vi "Write Serial Output Channel IO.vi"(0 "packet word":u8[](array[numeric]), 1 "reset":bool, 2 "resources":T1, 3 "filler valid":bool[](array[boolean]), 5 "end of packet":bool, 7 "generate packet":bool, 9 "input valid":bool, 11 "header valid":bool) -> (4 "ready to generate packet":bool, 6 "num packets in tx buffer":fxp<+,14,14>, 8 "num generated packets":u64, 14 "tready":bool)   [LabVIEW 2020, in "GettingStarted_Gen_148X_FPGA.lvlib"]
uses:
  GettingStarted_Gen_148X_FPGA.lvlib
  Types/Serial Output Channel Resources.ctl
  Common/Types/Serial Output Channel IO.ctl
  Common/Types/Serial Output Channel IO 32b.ctl
  Common/Types/Serial Output Channel IO 64b.ctl
  Common/Types/I2C IO.ctl
  Common/Types/Single Serial Channel Resources.ctl
  <vilib>/rvi/eio/common/nirviEmuTemplateMethod_errors.vi
  <instrlib>/_niInstr/Basic Elements/v1/FPGA/Private/Count Up U64.vi
  <instrlib>/_niInstr/Data Formatting/v1/FPGA/Private/Convert/U8 array to Boolean Array.vi
  <vilib>/eio/EIONode/EIONode.xnode
  <instrlib>/_niInstr/Data Formatting/v1/FPGA/niInstr Data Formatting v1 FPGA.lvlib
  <instrlib>/_niInstr/Basic Elements/v1/FPGA/niInstr Basic Elements v1 FPGA.lvlib
  Common/GettingStarted_Common_148X_FPGA.lvlib
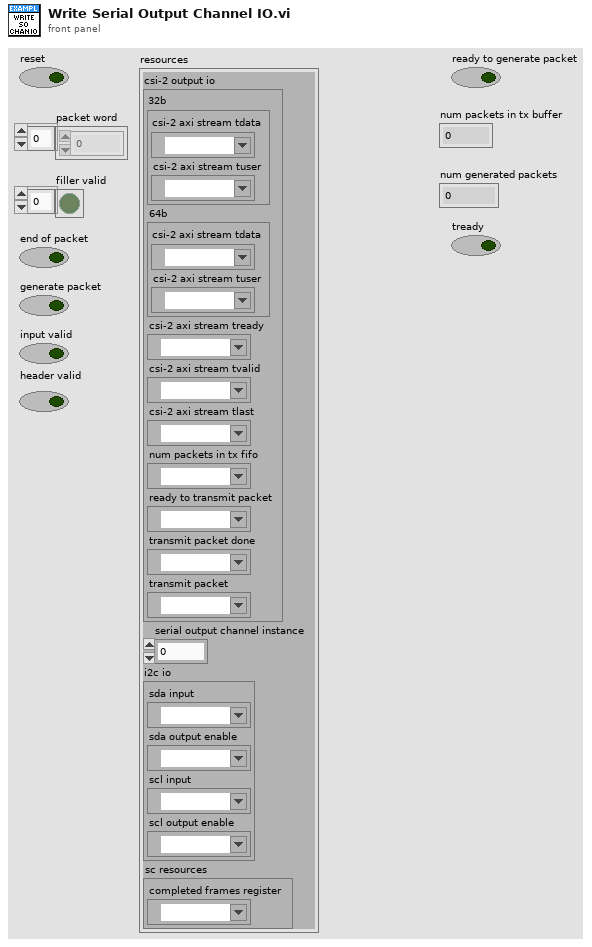
[diagram p1: front panel]
types:
  T1 = typedef "GettingStarted_Gen_148X_FPGA.lvlib/Serial Output Channel Resources.ctl" = cluster{"csi-2 output io":T2, "serial output channel instance":u8, "i2c io":T5, "sc resources":T6}
  T2 = typedef "GettingStarted_Common_148X_FPGA.lvlib/Serial Output Channel IO.ctl" = cluster{"32b":T3, "64b":T4, "csi-2 axi stream tready":refnum<k21>, "csi-2 axi stream tvalid":refnum<k21>, "csi-2 axi stream tlast":refnum<k21>, "num packets in tx fifo":refnum<k21>, "ready to transmit packet":refnum<k21>, "transmit packet done":refnum<k21>, "transmit packet":refnum<k21>}
  T3 = typedef "GettingStarted_Common_148X_FPGA.lvlib/Serial Output Channel IO 32b.ctl" = cluster{"csi-2 axi stream tdata":refnum<k21>, "csi-2 axi stream tuser":refnum<k21>}
  T4 = typedef "GettingStarted_Common_148X_FPGA.lvlib/Serial Output Channel IO 64b.ctl" = cluster{"csi-2 axi stream tdata":refnum<k21>, "csi-2 axi stream tuser":refnum<k21>}
  T5 = typedef "GettingStarted_Common_148X_FPGA.lvlib/I2C IO.ctl" = cluster{"sda input":refnum<k21>, "sda output enable":refnum<k21>, "scl input":refnum<k21>, "scl output enable":refnum<k21>}
  T6 = typedef "GettingStarted_Common_148X_FPGA.lvlib/Single Serial Channel Resources.ctl" = cluster{"completed frames register":refnum<k21>}
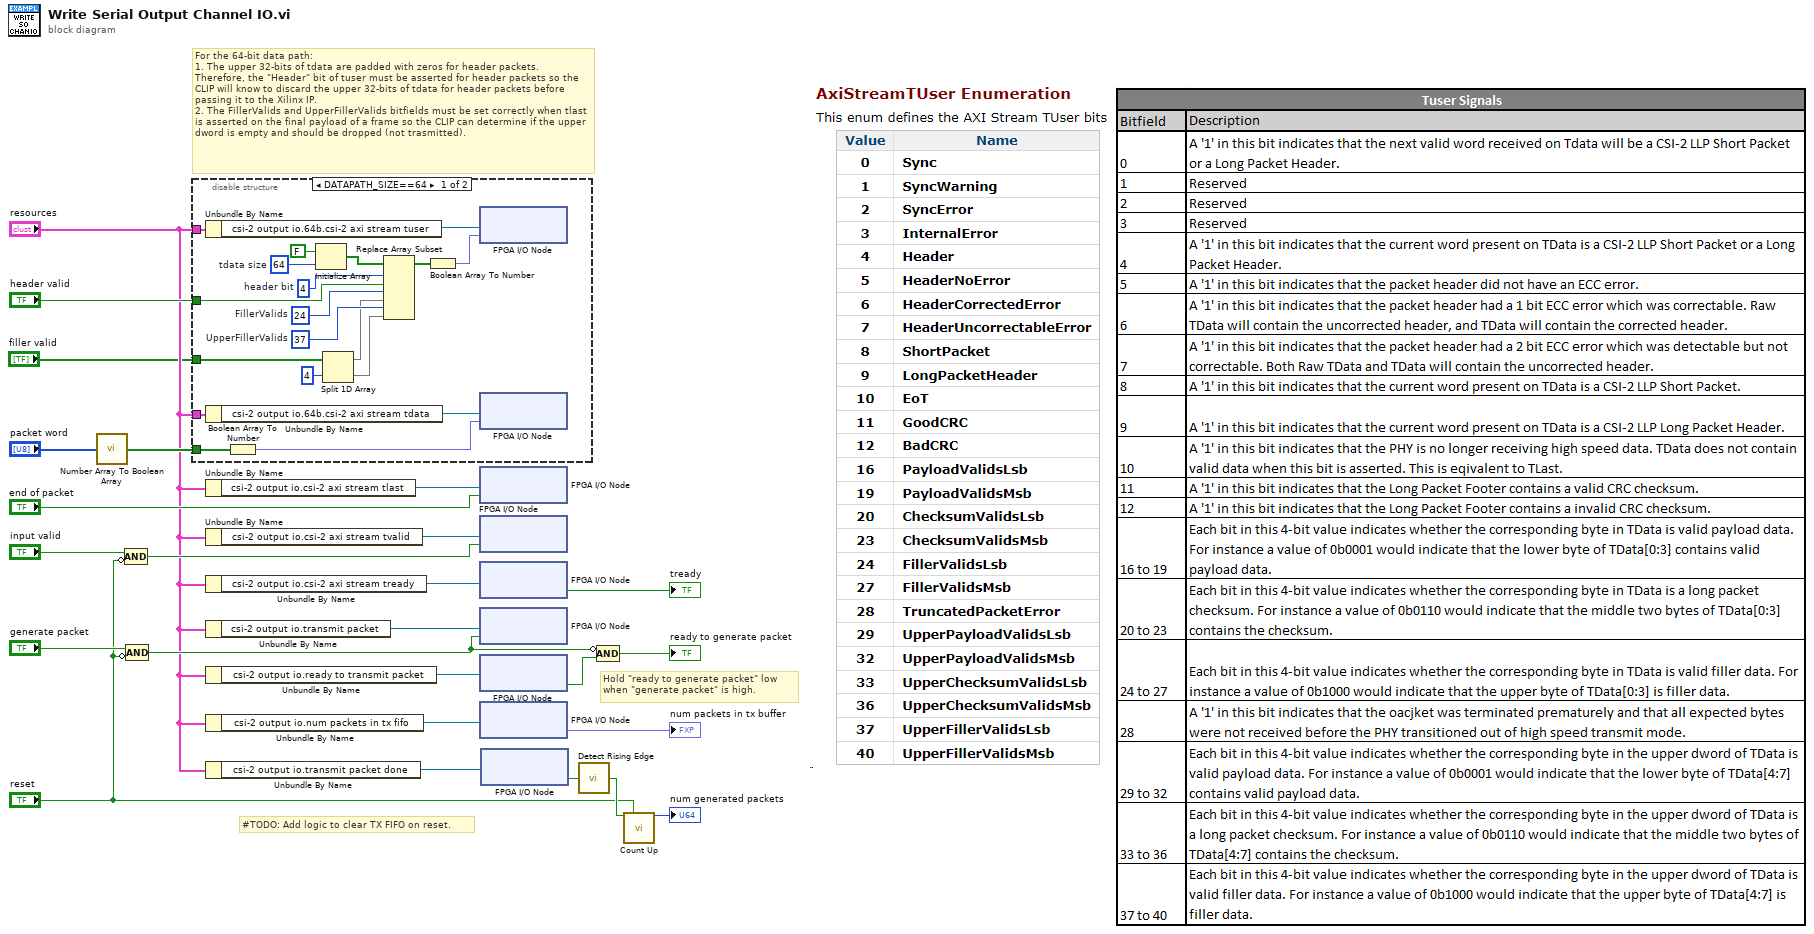
[diagram p0: block diagram]
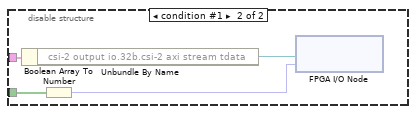
[diagram p2: hidden frame]
diagram:
  # "For the 64-bit data path:\n1. The upper 32-bits of tdata are padded with zeros for header packets.  Therefore, the \"Header\" bit of tuser must be asserted for header packets so the CLIP will know to discard the upper 32-bits of tdata for header packets before passing it to the Xilinx IP.\n2. The FillerValids and UpperFillerValids bitfields must be set correctly when tlast is asserted on the final payload of a frame so the CLIP can determine if the upper dword is empty and should be dropped (not trasmitted)."
  # "Hold \"ready to generate packet\" low \nwhen \"generate packet\" is high."
  # "#TODO: Add logic to clear TX FIFO on reset."
  n1 = call-poly <instrlib>:"Number Array To Boolean Array.vi"("data in"="packet word") -> ("data out"=w4:bool[])  [unwired: 14 in]
  n2 = Compound Arithmetic op=AND("input valid", invert "reset") -> (w9:bool)
  n3 = Compound Arithmetic op=AND("generate packet", invert "reset") -> (w7:bool)
  n4 = disable-structure shown="DATAPATH_SIZE==64" {
    disable-tunnel: "resources" -> [w34 w48]
    disable-tunnel: w4 -> [w43 w46]
    disable-tunnel: "header valid" -> [w37 _]
    disable-tunnel: "resources" -> [w32 _]
    disable-tunnel: "filler valid" -> [w29 _]
    frame condition #0 (active) {
      w30 = 37  # UpperFillerValids
      w31 = 24  # FillerValids
      w38 = 64  # tdata size
      w39 = 4  # header bit
      n5 = Unbundle By Name(w32) -> ("csi-2 output io.64b.csi-2 axi stream tuser"=w33:refnum<k21>)
      n6 = Unbundle By Name(w34) -> ("csi-2 output io.64b.csi-2 axi stream tdata"=w44:refnum<k21>)
      n7 = Boolean Array To Number(Boolean array=w43) -> (number=w42:fxp<+,64,64>)
      n8 = Initialize Array(FALSE, w38) -> (w40:bool[])
      n9 = Split 1D Array(array=w29, index=4) -> (first subarray=w27:bool[], second subarray=w26:bool[])
      n10 = Replace Array Subset(array=w40, new element #1=w37, index #1=w39, new element #2=w27, index #2=w31, new element #3=w26, index #3=w30) -> (w36:bool[])
      n11 = Boolean Array To Number(Boolean array=w36) -> (number=w35:fxp<+,64,64>)
      n12 = xnode "FPGA I/O Node"("I/O Item"=w35, "FPGA I/O In"=w33) -> ()  [unwired: 1 out]
      n13 = xnode "FPGA I/O Node"("I/O Item"=w42, "FPGA I/O In"=w44) -> ()  [unwired: 1 out]
    }
    frame condition #1 {
      n14 = Unbundle By Name(w48) -> ("csi-2 output io.32b.csi-2 axi stream tdata"=w47:refnum<k21>)
      n15 = Boolean Array To Number(Boolean array=w46) -> (number=w45:fxp<+,32,32>)
      n16 = xnode "FPGA I/O Node"("I/O Item"=w45, "FPGA I/O In"=w47) -> ()  [unwired: 1 out]
    }
  }
  n17 = Unbundle By Name("resources") -> ("csi-2 output io.csi-2 axi stream tlast"=w24:refnum<k21>)
  n18 = Unbundle By Name("resources") -> ("csi-2 output io.csi-2 axi stream tvalid"=w22:refnum<k21>)
  n19 = Unbundle By Name("resources") -> ("csi-2 output io.csi-2 axi stream tready"=w21:refnum<k21>)
  n20 = Unbundle By Name("resources") -> ("csi-2 output io.transmit packet"=w19:refnum<k21>)
  n21 = Unbundle By Name("resources") -> ("csi-2 output io.ready to transmit packet"=w18:refnum<k21>)
  n22 = Unbundle By Name("resources") -> ("csi-2 output io.num packets in tx fifo"=w17:refnum<k21>)
  n23 = Unbundle By Name("resources") -> ("csi-2 output io.transmit packet done"=w15:refnum<k21>)
  n24 = xnode "FPGA I/O Node"("I/O Item"="end of packet", "FPGA I/O In"=w24) -> ()  [unwired: 1 out]
  n25 = xnode "FPGA I/O Node"("I/O Item"=w9, "FPGA I/O In"=w22) -> ()  [unwired: 1 out]
  n26 = xnode "FPGA I/O Node"("FPGA I/O In"=w21) -> ("I/O Item"=→"tready":bool)  [unwired: 1 out]
  n27 = xnode "FPGA I/O Node"("I/O Item"=w7, "FPGA I/O In"=w19) -> ()  [unwired: 1 out]
  n28 = xnode "FPGA I/O Node"("FPGA I/O In"=w18) -> ("I/O Item"=w6:bool)  [unwired: 1 out]
  n29 = xnode "FPGA I/O Node"("FPGA I/O In"=w17) -> ("I/O Item"=→"num packets in tx buffer":fxp<+,14,14>)  [unwired: 1 out]
  n30 = xnode "FPGA I/O Node"("FPGA I/O In"=w15) -> ("I/O Item"=w13:bool)  [unwired: 1 out]
  n31 = call <instrlib>:"Detect Rising Edge.vi"("signal"=w13) -> ("edge detected"=w14:bool)  [unwired: 14 in]
  n32 = Compound Arithmetic op=AND(invert w7, w6) -> (→"ready to generate packet":bool)
  n33 = call-poly <instrlib>:"Count Up.vi"("increment"=w14, "reset"="reset") -> ("count out"=→"num generated packets":u64)  [unwired: 13 in]
